vi "Read_Wrap.vi"(2 "Value":T1, 8 "error in (no error)":errorcluster, 11 "Var_DBL in":refnum<class "Var_Bool.lvclass">) -> (0 "error out":errorcluster, 3 "Var_DBL out":refnum<class "Var_Bool.lvclass">)   [LabVIEW 2021, in "Var_Bool.lvclass"]
uses:
  Var_Bool.lvclass
  Var_Bool.lvclass/Var_Bool.ctl
  Type.ctl
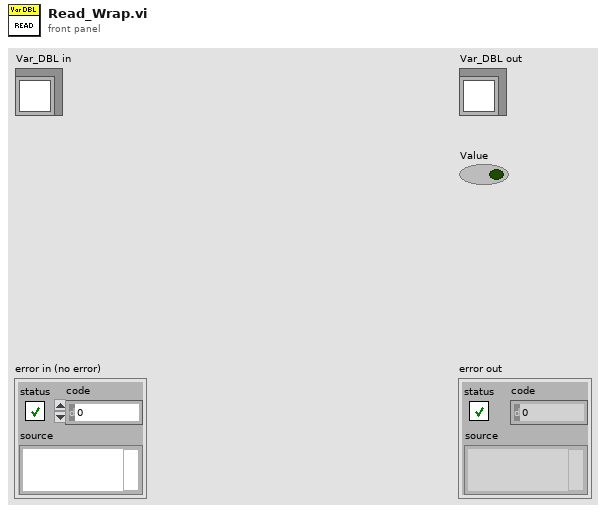
[diagram p1: front panel]
types:
  T1 = typedef "Var_Bool.lvclass/Type.ctl" = bool
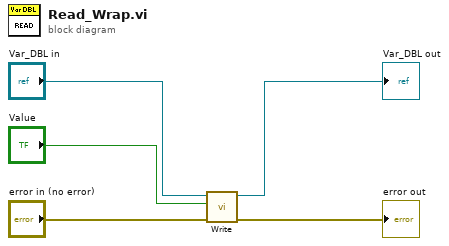
[diagram p0: block diagram]
diagram:
  n1 = call-dynamic "Write.vi"("error in (no error)"="error in (no error)", "Value"="Value", "Double Float.lvclass_340760 in"="Var_DBL in") -> ("error out"=→"error out":errorcluster, "Double Float.lvclass_340760 out"=→"Var_DBL out":refnum<class "Var_Bool.lvclass">)  [unwired: 7 in]
